vi "Multiply - RM,RM.vi"(1 "Real Matrix B":T1, 2 "Real Matrix A":T1) -> (0 "A * B":T1)   [LabVIEW 2020, in "NI_Matrix.lvlib"]
doc: "Returns the product of the inputs."
uses:
  NI_Matrix.lvlib
  RealMatrix.ctl
  Real A x B.vi
  NI_AALBase.lvlib
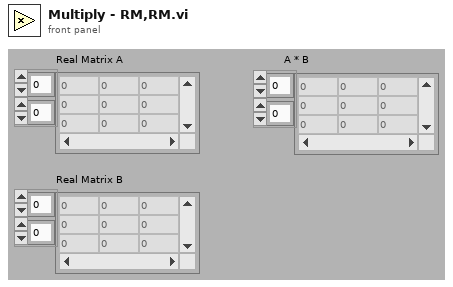
[diagram p1: front panel]
types:
  T1 = typedef "NI_Matrix.lvlib/RealMatrix.ctl" = dbl[][]
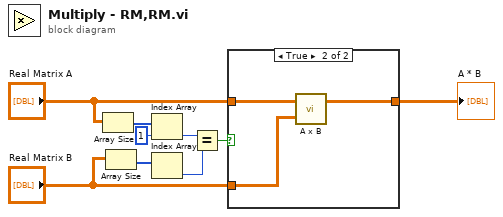
[diagram p0: block diagram]
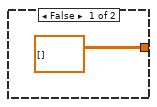
[diagram p2: hidden frame]
diagram:
  n1 = Array Size(array="Real Matrix A") -> (size(s)=w5:i32[])
  n2 = Array Size(array="Real Matrix B") -> (size(s)=w6:i32[])
  n3 = Index Array(array=w5, index=1) -> (element=w8:i32)
  n4 = Index Array(array=w6) -> (element=w4:i32)  [unwired: 1 in]
  n5 = Equal?(x=w8, y=w4) -> (x = y?=w1:bool)
  n6 = case shown="True" w1 {
    tunnel: "Real Matrix A" -> [_ w13]
    tunnel: "Real Matrix B" -> [_ w11]
    tunnel: [T1 [] ("A + B") w12] -> w9
    frame False {
    }
    frame True {
      n7 = call-poly "A x B.vi"("B"=w11, "A"=w13) -> ("A x B"=w12:T1)  [unwired: 1 out]
    }
  }
  "A * B" <- w9
